vi "View Complex Impedance.vi"() -> ()   [LabVIEW 2016]
panel:
  in  "Tab Control 2":T1(tab)
  out "Magnitude":cluster{"Y":dbl[], "Y":dbl[]}[](graph)
  out "Phase":cluster{"Y":dbl[], "Y":dbl[]}[](graph)
  out "Magnitude":cluster{"Y":dbl[], "Y":dbl[]}[](graph)
  out "Phase":cluster{"Y":dbl[], "Y":dbl[]}[](graph)
  out "Magnitude 2":cluster{"Y":dbl[], "Y":dbl[]}[](graph)
  out "Phase 2":cluster{"Y":dbl[], "Y":dbl[]}[](graph)
  in  "Tab Control":enum32{"Lockin  1", "Lockin 2", "Temp"}(tab)
  in  "X":cluster{"Y":dbl[], "Y":dbl[]}[](graph)
  in  "Y":cluster{"Y":dbl[], "Y":dbl[]}[](graph)
  in  "X 3":cluster{"Y":dbl[], "Y":dbl[]}[](graph)
  in  "Y 4":cluster{"Y":dbl[], "Y":dbl[]}[](graph)
  out "Temp vs Time":cluster{"Y":dbl[], "Y":dbl[]}[](graph)
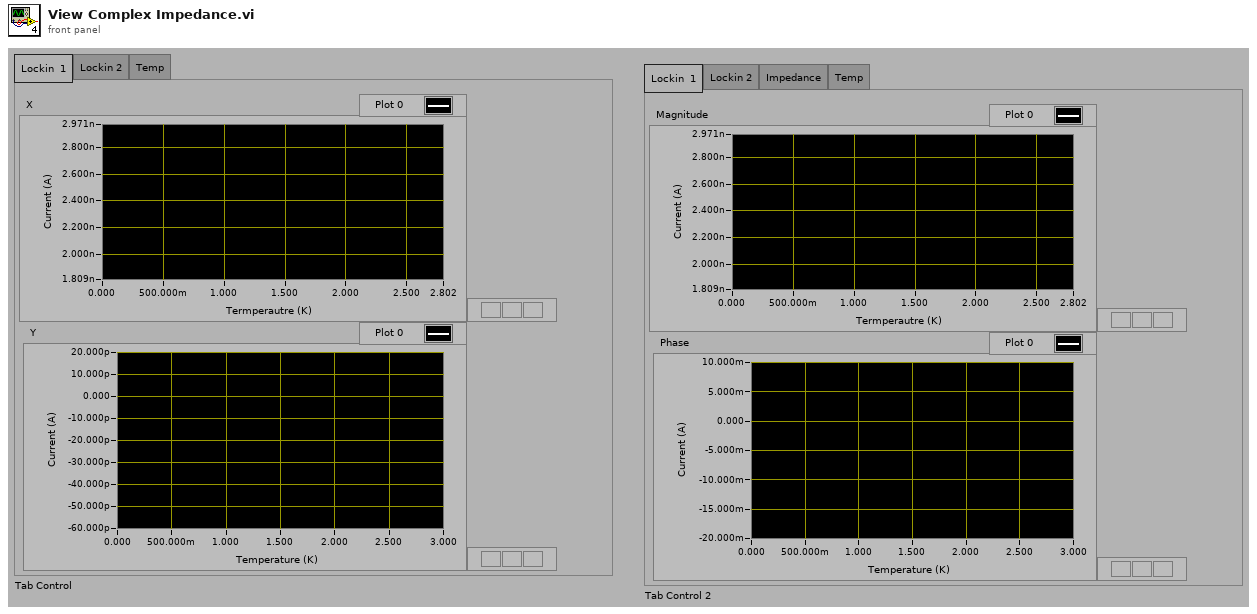
[diagram p1: front panel]
types:
  T1 = enum32{"Lockin  1", "Lockin 2", "Impedance", "Temp"}
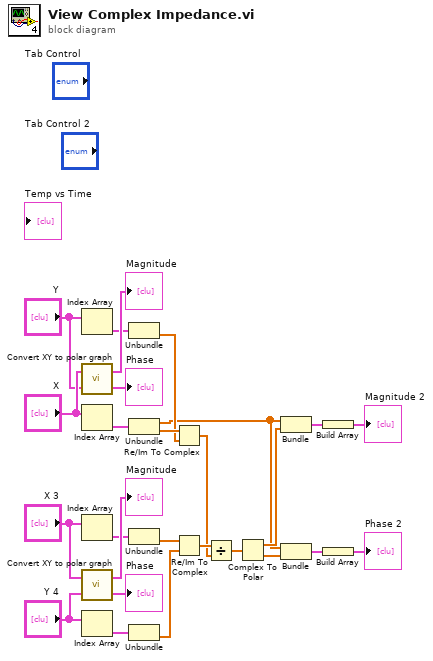
[diagram p0: block diagram]
diagram:
  n1 = Index Array(array="Y") -> (element=w22:cluster{"Y":dbl[], "Y":dbl[]})  [unwired: 1 in]
  n2 = call "Convert XY to polar graph.vi"("Y"="Y", "X"="X") -> ("Array"=→"Phase":cluster{"Y":dbl[], dbl[]}[], "Array 2"=→"Magnitude":cluster{"Y":dbl[], dbl[]}[])
  n3 = Index Array(array="X") -> (element=w21:cluster{"Y":dbl[], "Y":dbl[]})  [unwired: 1 in]
  n4 = Index Array(array="X 3") -> (element=w14:cluster{"Y":dbl[], "Y":dbl[]})  [unwired: 1 in]
  n5 = call "Convert XY to polar graph.vi"("Y"="Y 4", "X"="X 3") -> ("Array"=→"Phase":cluster{"Y":dbl[], dbl[]}[], "Array 2"=→"Magnitude":cluster{"Y":dbl[], dbl[]}[])
  n6 = Index Array(array="Y 4") -> (element=w13:cluster{"Y":dbl[], "Y":dbl[]})  [unwired: 1 in]
  n7 = Unbundle(w22) -> ("Y"=w17:dbl[])  [unwired: 1 out]
  n8 = Unbundle(w21) -> ("Y"=w3:dbl[], "Y"=w18:dbl[])
  n9 = Unbundle(w14) -> ("Y"=w15:dbl[])  [unwired: 1 out]
  n10 = Unbundle(w13) -> ("Y"=w16:dbl[])  [unwired: 1 out]
  n11 = Re/Im To Complex(1:w17, 2:w18) -> (0:w9:cdb[])
  n12 = Re/Im To Complex(1:w16, 2:w15) -> (0:w10:cdb[])
  n13 = Divide(x=w10, y=w9) -> (x/y=w6:cdb[])
  n14 = Complex To Polar(r * e^(i*theta)=w6) -> (r=w5:dbl[], theta=w4:dbl[])
  n15 = Bundle("Y"=w3, w5) -> (w7:cluster{"Y":dbl[], dbl[]})  [unwired: 1 in]
  n16 = Bundle("Y"=w3, w4) -> (w8:cluster{"Y":dbl[], dbl[]})  [unwired: 1 in]
  n17 = Build Array(w7) -> (→"Magnitude 2":cluster{"Y":dbl[], dbl[]}[])
  n18 = Build Array(w8) -> (→"Phase 2":cluster{"Y":dbl[], dbl[]}[])
